vi "First-Order Hold (DBL).vi"(2 "initialize":bool, 3 "hold time in cycles":i32, 5 "input point":dbl format="%.2f") -> (1 "output point":dbl format="%.2f")   [LabVIEW 2017, in "NI_AdvCtrl_discrete linear.lvlib"]
doc: "LabVIEW no longer supports this VI. You can obtain similar functionality by installing the LabVIEW Simulation Module.\n\nA first-order sample and hold predicts the value of the output based on the first derivative of a given input signal."
uses:
  <vilib>/addons/control/advanced/NI_AdvCtrl_discrete linear.lvlib
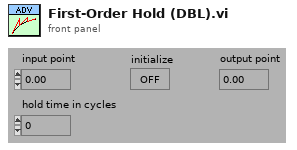
[diagram p1: front panel]
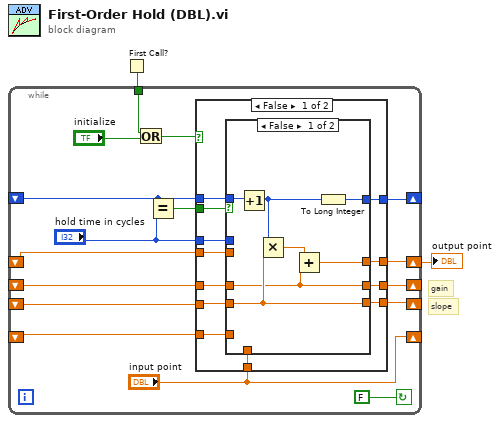
[diagram p0: block diagram]
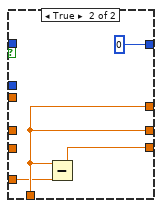
[diagram p2: hidden frame]
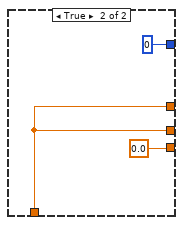
[diagram p3: hidden frame]
diagram:
  # "gain"
  # "slope"
  n1 = First Call?() -> (First Call?: T/F=w1:bool)
  n2 = while {
    tunnel: w1 -> [w4]
    shift-left: _ -> [w7]
    shift-right: [w10] -> _
    shift-left: _ -> [w12]
    shift-right: [w11] -> _
    shift-left: _ -> [w13]
    shift-right: [w14] -> _
    shift-left: _ -> [w16]
    shift-right: [w18] -> w2
    shift-left: _ -> [w17]
    shift-right: ["input point"] -> _
    stop <- FALSE continue-if-true
    n3 = Or(x=w4, y="initialize") -> (x .or. y?=w3:bool)
    n4 = Equal?(x=w7, y="hold time in cycles") -> (x = y?=w8:bool)
    n5 = case shown="False" w3 {
      tunnel: "input point" -> [w30 w44]
      tunnel: [w29 w44] -> w18
      tunnel: w17 -> [w28 _]
      tunnel: w16 -> [w27 _]
      tunnel: [w26 w44] -> w14
      tunnel: w13 -> [w25 _]
      tunnel: w12 -> [w23 _]
      tunnel: [w24 0.0] -> w11
      tunnel: "hold time in cycles" -> [w22 _]
      tunnel: [w19 0] -> w10
      tunnel: w8 -> [w21 _]
      tunnel: w7 -> [w20 _]
      frame False {
        n6 = case shown="False" w21 {
          tunnel: [w34 w41] -> w29
          tunnel: w30 -> [_ w41]
          tunnel: w28 -> [_ w40]
          tunnel: w27 -> [_ _]
          tunnel: [w36 w41] -> w26
          tunnel: w25 -> [w36 _]
          tunnel: [w37 w39] -> w24
          tunnel: w23 -> [w37 _]
          tunnel: w22 -> [_ _]
          tunnel: w20 -> [w33 _]
          tunnel: [w32 0] -> w19
          frame False {
            n7 = Increment(x=w33) -> (x+1=w31:i32)
            n8 = Multiply(x=w31, y=w37) -> (x*y=w35:dbl)
            n9 = Add(x=w35, y=w36) -> (x+y=w34:dbl)
            n10 = To Long Integer(number=w31) -> (32bit integer=w32:i32)
          }
          frame True {
            n11 = Subtract(x=w41, y=w40) -> (x-y=w39:dbl)
          }
        }
      }
      frame True {
      }
    }
  }
  "output point" <- w2
